vi "Evaluate.vi"(7 "Message (\"\")":string, 8 "error in (no error)":errorcluster, 10 "Actual":variant, 11 "Constraint in":refnum<class "Constraint.lvclass">) -> (0 "error out":errorcluster, 3 "Constraint out":refnum<class "Constraint.lvclass">)   [LabVIEW 2017, in "Constraint.lvlib" / "Constraint.lvclass"]
doc: "Evaluates the constraint for <B>Actual</B>."
uses:
  Constraint.lvclass
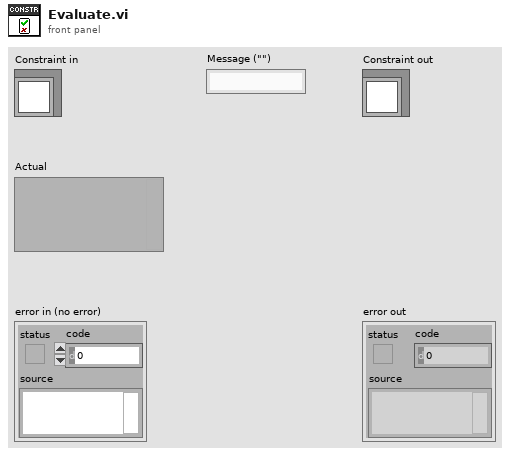
[diagram p1: front panel]
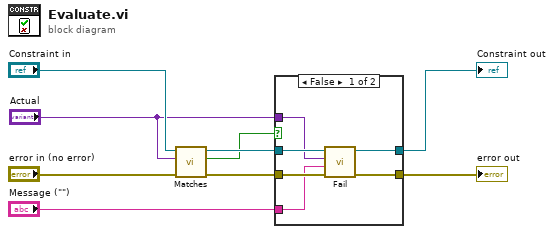
[diagram p0: block diagram]
diagram:
  n1 = call-dynamic "Matches.vi"("error in (no error)"="error in (no error)", "Actual"="Actual", "Constraint in"="Constraint in") -> ("error out"=w3:errorcluster, "Result"=w1:bool, "Constraint out"=w2:refnum<class "Constraint.lvclass">)  [unwired: 6 in]
  n2 = case shown="False" w1 {
    tunnel: w3 -> [w15 w16]
    tunnel: [w14 w16] -> w8
    tunnel: "Actual" -> [w10 _]
    tunnel: w2 -> [w13 w17]
    tunnel: [w12 w17] -> w6
    tunnel: "Message (\"\")" -> [w11 _]
    frame False {
      n3 = call-dynamic "Fail.vi"("error in (no error)"=w15, "Message (\"\")"=w11, "Actual"=w10, "Constraint in"=w13) -> ("error out"=w14:errorcluster, "Constraint out"=w12:refnum<class "Constraint.lvclass">)  [unwired: 6 in]
    }
    frame True {
    }
  }
  "error out" <- w8
  "Constraint out" <- w6
